vi "CRYData View Graph Get.vi"(11 "Queue Name":string) -> (3 "Flattened Graph ViewPro":string)   [LabVIEW 2013]
uses:
  Control/CRYGraph Property.ctl
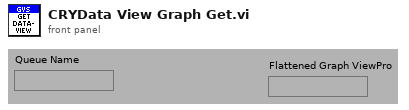
[diagram p1: front panel]
types:
  T1 = typedef "CRYGraph Property.ctl" = cluster{"LegendShow":bool, "Legend Splitter Position":dbl, "Data Names":string[], "Item Symbols":i32[], "Color Array":u32[], "Flattened Plot Property":string, "CursorShow":bool, "Flattened Cursor Property":string, "Graph Number":i32, "Flattened Scale Property":string, "PreviewShow":bool, "MagnitudeShow":bool, "PaletteShow":bool, "XYShow":bool, "FrequencyShow":bool, "Frequency Splitter Position":dbl, "XYGraph Splitter Position":dbl, "Frequency Symbols":i32[], "LegendVScrollShow":bool, "FrequencyVScrollShow":bool, "PhaseShow":bool, "Title Name":string}
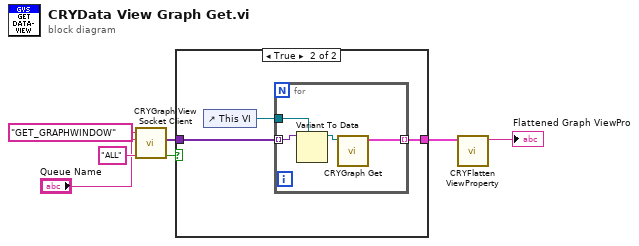
[diagram p0: block diagram]
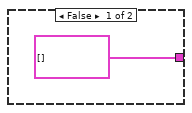
[diagram p2: hidden frame]
diagram:
  n1 = call "CRYGraph View Socket Client.vi"("sOption"="ALL", "sData"="Queue Name", "sAction"="GET_GRAPHWINDOW") -> ("bResult Out"=w3:bool, "Variant Out"=w4:variant[])  [unwired: 5 in, 2 out]
  n2 = case shown="True" w3 {
    tunnel: w4 -> [_ w11]
    tunnel: [T1[] [] w10] -> w1
    frame False {
    }
    frame True {
      n3 = control-ref of="This VI"() -> (w9:refnum<vi>)
      n4 = for {
        tunnel: w11 -> [w15] mode=indexing
        tunnel: [w13] -> w10 mode=indexing
        tunnel: w9 -> [w12]
        n5 = Variant To Data(type=w12, Variant=w15) -> (data=w14:refnum<vi>)  [unwired: 1 in, 1 out]
        n6 = call "CRYGraph Get.vi"("pGraph VI In"=w14) -> ("Graph Cluster"=w13:T1)  [unwired: 10 in]
      }
    }
  }
  n7 = call "CRYFlatten ViewProperty.vi"("GraphViewProperty"=w1) -> ("ViewPro flattened"=→"Flattened Graph ViewPro":string)  [unwired: 10 in]
